vi "download.vi"(8 "error in (no error)":errorcluster, 10 "target_path":path, 11 "address":string) -> (0 "error out":errorcluster)   [LabVIEW 2015, in "lv-bin-wget.lvlib" / "v1.lvlib"]
uses:
  v1.lvlib
  <userlib>/antonio-alexander/lv-bin/lv-bin/public/api/v1/v1.lvlib
  lv-bin-wget.lvlib
panel:
  in  "quiet?":bool=TRUE
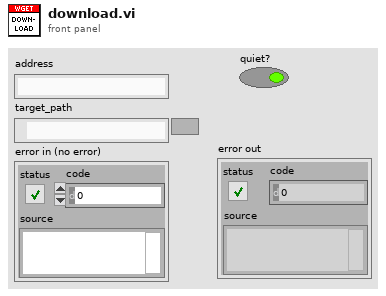
[diagram p1: front panel]
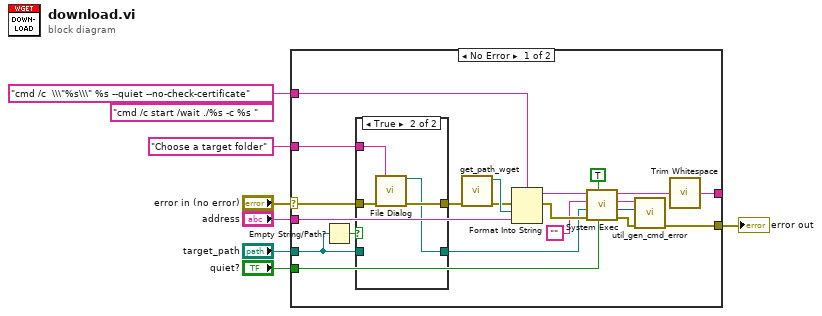
[diagram p0: block diagram]
diagram:
  (unwired) "cmd /c start /wait ./%s -c %s " ("format string")
  n1 = case shown="No Error" "error in (no error)" {
    selector: "error in (no error)" -> [w24 w35]
    tunnel: [w19 w35] -> w6
    tunnel: "target_path" -> [w23 _]
    tunnel: "Choose a target folder" ("prompt") -> [w21 _]
    tunnel: "quiet?" -> [w18 _]
    tunnel: [w14 _] -> _
    tunnel: "address" -> [w12 _]
    tunnel: "cmd /c  \\\"%s\\\" %s --quiet --no-check-certificate" ("format string") -> [w13 _]
    frame No Error {
      n2 = Empty String/Path?(string/path=w23) -> (empty?=w22:bool)
      n3 = case shown="True" w22 {
        tunnel: w24 -> [w29 w34]
        tunnel: [w29 w33] -> w10
        tunnel: w23 -> [w30 _]
        tunnel: w21 -> [_ w32]
        tunnel: [w30 w31] -> w8
        frame False {
        }
        frame True {
          n4 = call "File Dialog"("prompt"=w32, "error in"=w34) -> ("selected path"=w31:path, "error out"=w33:errorcluster)  [unwired: 10 in, 2 out]
        }
      }
      n5 = call "get_path_wget.vi"("error in (no error)"=w10) -> ("error out"=w9:errorcluster, "wget"=w11:path)  [unwired: 9 in]
      n6 = Format Into String(format string=w13, error in=w9, w11, w12) -> (resulting string=w27:string, error out=w28:errorcluster)  [unwired: 1 in]
      n7 = call <vilib>:"System Exec.vi"("run minimized? (F)"=w18, "wait until completion? (T)"=TRUE, "error in (no error)"=w28, "working directory"=w8, "standard input"="", "command line"=w27) -> ("error out"=w20:errorcluster, "return code"=w15:i32, "standard error"=w17:string, "standard output"=w16:string)  [unwired: 2 in]
      n8 = call <userlib>:"util_gen_cmd_error.vi"("error in (no error)"=w20, "return_code"=w15, "standard_error"=w17) -> ("error out"=w19:errorcluster)  [unwired: 8 in]
      n9 = call <vilib>:"Trim Whitespace.vi"("string"=w16) -> ("trimmed string"=w14:string)  [unwired: 1 in]
    }
    frame Error {
    }
  }
  "error out" <- w6
